vi "sub_tcpbuf_fgv.vi"(7 "cmd":enum16{"ini", "add", "use", "check"}(ring), 8 "error in":errorcluster, 10 "exit":bool, 11 "cmd_str":string) -> (0 "error out":errorcluster, 2 "data exist":bool, 3 "element":string)   [LabVIEW 2018]
panel:
  out "size(s)":i32
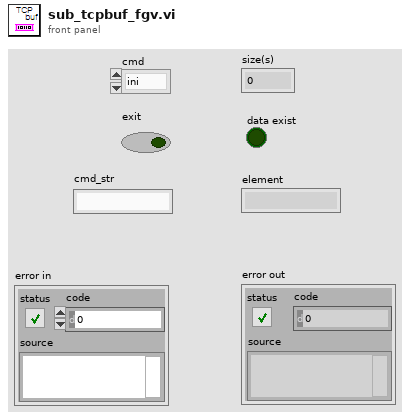
[diagram p1: front panel]
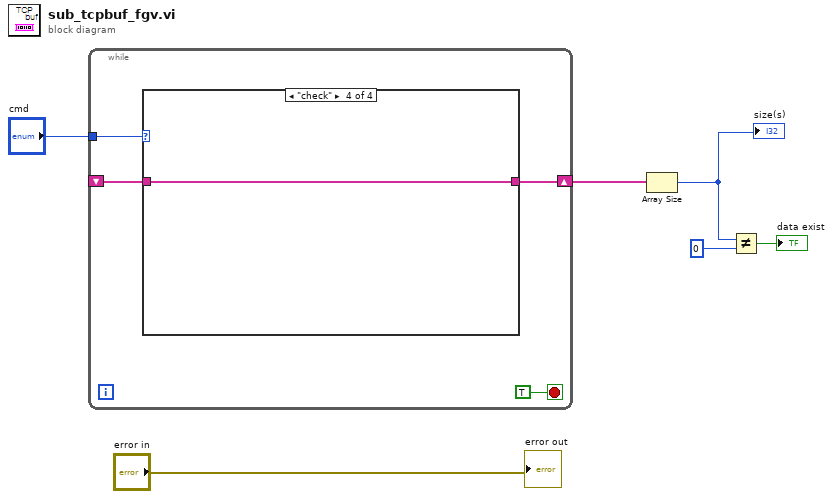
[diagram p0: block diagram]
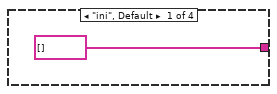
[diagram p2: hidden frame]
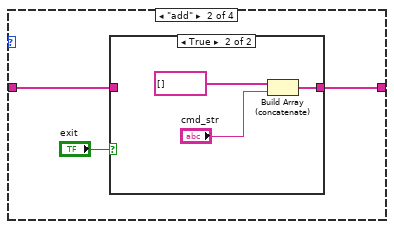
[diagram p3: hidden frame]
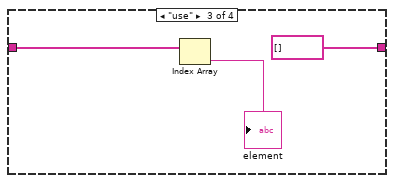
[diagram p5: hidden frame]
diagram:
  n1 = while {
    tunnel: "cmd" -> [w9]
    shift-right: [w7] -> w4
    shift-left: _ -> [w8]
    stop <- TRUE stop-if-true
    n2 = case shown="\"check\"" w9 {
      tunnel: w8 -> [_ w12 w21 w22]
      tunnel: [string[] [] w14 string[] [] w22] -> w7
      frame "ini", Default {
      }
      frame "add" {
        n3 = case shown="True" "exit" {
          tunnel: [w15 w17] -> w14
          tunnel: w12 -> [w15 _]
          frame False {
          }
          frame True {
            n4 = Build Array (concatenate)(string[] [], "cmd_str") -> (w17:string[])
          }
        }
      }
      frame "use" {
        n5 = Index Array(array=w21) -> (element=→"element":string)  [unwired: 1 in]
      }
      frame "check" {
      }
    }
  }
  n6 = Array Size(array=w4) -> (size(s)=w3:i32)
  "size(s)" <- w3
  n7 = Not Equal?(x=w3, y=0) -> (x != y?=→"data exist":bool)
  "error out" <- "error in"
